vi "8-Tap 8-bit Camera with DRAM no Serial or Packing V4(FPGA).vi"() -> ()   [LabVIEW 2013]
doc: "This is the FPGA VI for the 10-Tap 8-Bit Camera with DRAM example. This example demonstrates how to acquire images from a 10-tap, 8-bit, extended configuration, Camera Link camera and transfer the images to the host. This example supports area scan and line scan cameras for both continuous and finite acquisitions.\n\nThis example also demonstrates the use of DRAM as a frame buffer for very high speed acquisitions. Data packing and flow-control are also employed to maximize use of the available DRAM and FIFOs in terms of both memory space and performance.\n\nAdditionally, the example demonstrates the serial server, which allows third-party camera configuration utilities to communicate with the camera using the Camera Link serial interface while this VI is running."
uses:
  <vilib>/rvi/DataTransferAndStorage/Container/XNode/niFpgaContainer.xnode
  <vilib>/Platform/TimedLoop/XDataNode/XDataNode.xnode
  <vilib>/Platform/TimedLoop/XDataNode/timing_clust.ctl
  <vilib>/Platform/TimedLoop/XDataNode/XDNodeRunTimeDep.lvlib
  <vilib>/Platform/TimedLoop/XDataNode/wakeup.ctl
  <vilib>/Platform/TimedLoop/XDataNode/nitl_modes.ctl
  <vilib>/eio/EIONode/EIONode.xnode
  <vilib>/rvi/eio/common/nirviEmuTemplateMethod_errors.vi
  <vilib>/rvi/FIFO/Fifo_Resource/nirvififoEmulationGetNumberOfElementsToRead.vi
  <vilib>/rvi/interface/RandomDataEmulation/nirviRandomDataFpgaReadWriteTemplate.vi
  <vilib>/rvi/FIFO/Fifo_Resource/nirvififoEmulationRead.vi
  <vilib>/rvi/FIFO/Fifo_Resource/nirvififoEmulationWrite.vi
  FPGA/Globals/Accumulated Sector Intensity.vi
  FPGA/Globals/Pixel Location Global.vi
  FPGA/Globals/Sector Parameter Global.vi
  <vilib>/rvi/FIFO/Fifo_Resource/nirvififoEmulationGetNumberOfElementsToWrite.vi
  Common/CL Data to Pixels/8 Tap 8-Bit.vi
  Common/CL Signal Mapping.ctl
  Common/CL Configuration.ctl
  FPGA/Sector/Accumulate/Sector Parameter Cluster.ctl
panel:
  in  "Right End Angle Duty Cycle":fxp<+,8,0>
  in  "Right Start Angle Duty Cycle":fxp<+,8,0>
  in  "Left End Angle Duty Cycle":fxp<+,8,0>
  in  "Left Start Angle Duty Cycle":fxp<+,8,0>
  in  "X Resolution":u16=1000
  in  "Y Resolution":u16=1000
  out "Analysis Ticks":u32
  out "Right Sector Edge":u8
  out "Left Sector Edge":u8
  in  "[Average BG Intensity]":u8[](array[numeric])=[0, 0, 0, 0, 0, 0, 0, 0, 0, 0, 0, 0, 0, 0, 0, 0, 0, 0, 0, 0, 0, 0, 0, 0, 0, 0, 0, 0, 0, 0, 0, 0]
  in  "Sector Threshold":u8
  in  "# of Frames to Average":u8
  in  "Sector Parameters Right":T1={"Start Angle"=0.0, "End Angle"=0.4708251953125, "Inner Radius"=309, "Outter Radius"=405, "Hinge X"=685, "Hinge Y"=527, "NumWingSectors"=8}
  in  "Sector Parameters Left":T1={"Start Angle"=0.65740966796875, "End Angle"=0.99468994140625, "Inner Radius"=309, "Outter Radius"=405, "Hinge X"=464, "Hinge Y"=534, "NumWingSectors"=8}
  in  "CL Config.Configuration":T2=enum."Full"
  in  "CL Config.Signal Mapping":T3=enum."Basler 10-tap"
  in  "CL Config.Line Scan":bool
  in  "CL Config.DVAL Active High":bool=TRUE
  in  "CL Config.LVAL Active High":bool=TRUE
  in  "CL Config.FVAL Active High":bool=TRUE
  in  "CL Config.Spare Active High":bool=TRUE
  in  "Acq Control.Line Scan Height":u32
  in  "Acq Control.Frames To Acq":u32
  in  "Acq Control.Acquire":bool
  in  "Acq Control.Cancel Acq":bool
  in  "Acq Control.Ignore DVAL":bool
  in  "Acq Control.Initialize":bool
  out "Acq Status.Acq In Progress":bool
  out "Acq Status.Clocks Per Line":u32
  out "Acq Status.Frames Acq'd":u32
  out "Acq Status.Lines Per Frame":u32
  out "Acq Status.DMA Write Timeout":bool
  out "Acq Status.Initialized":bool
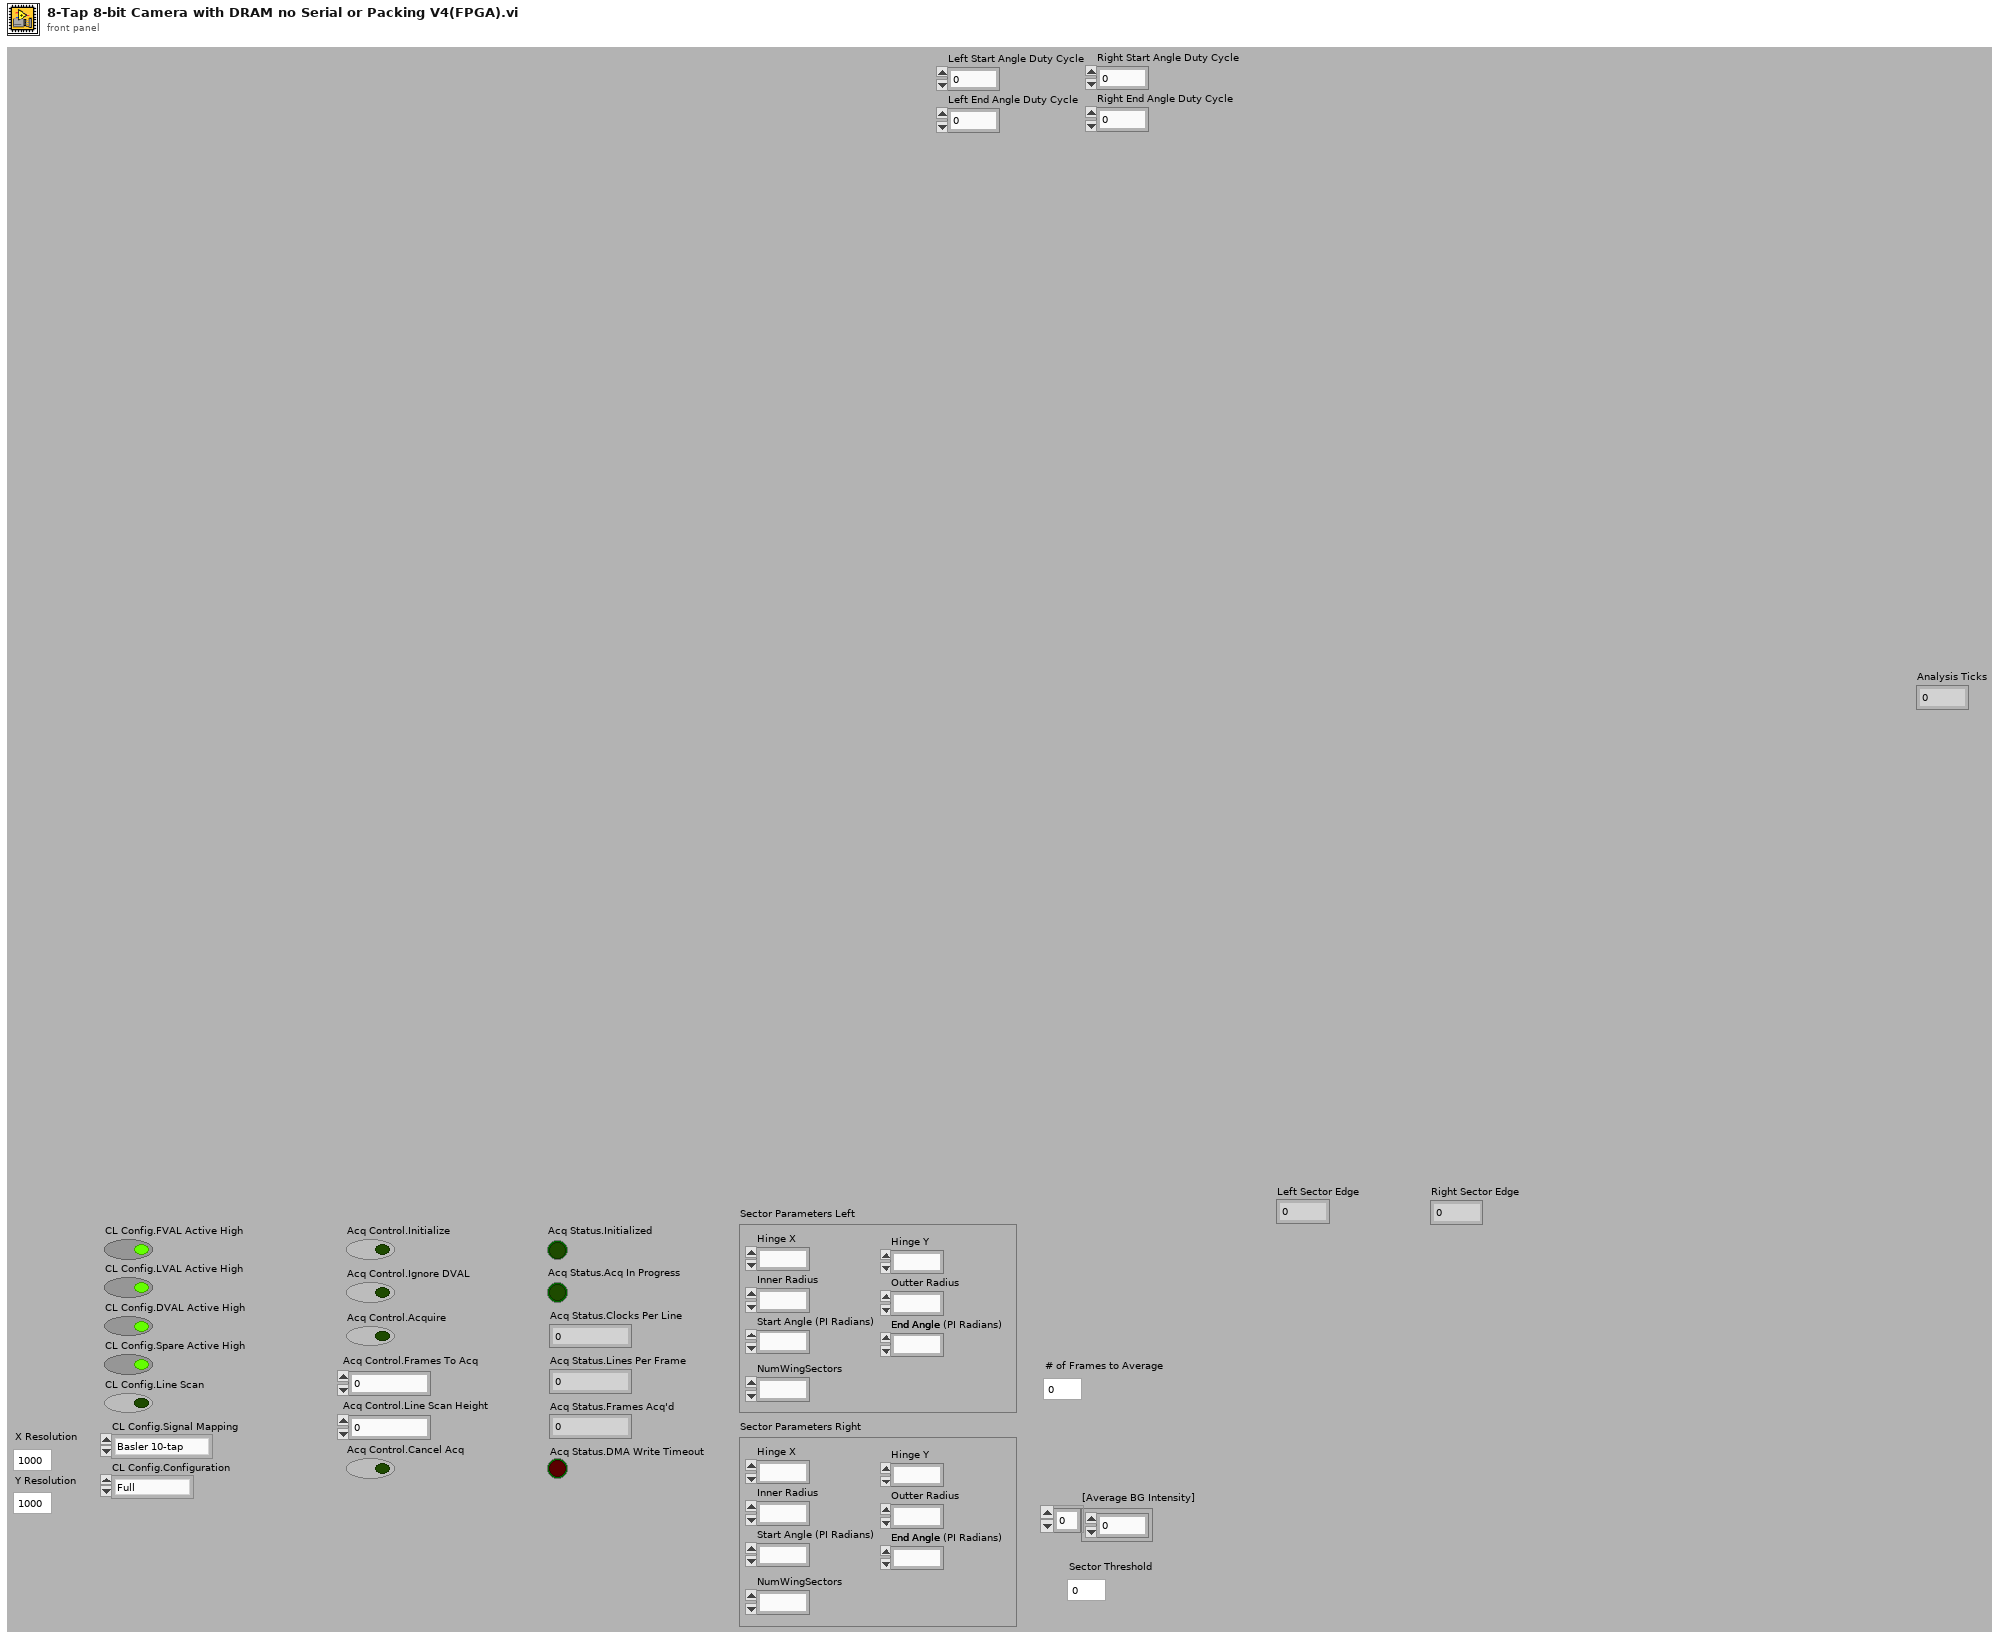
[diagram p1: front panel]
types:
  T1 = typedef "Sector Parameter Cluster.ctl" = cluster{"Start Angle":fxp<+/-,17,2>, "End Angle":fxp<+,17,3>, "Inner Radius":u16, "Outter Radius":u16, "Hinge X":u16, "Hinge Y":u16, "NumWingSectors":u8}
  T2 = typedef "CL Configuration.ctl" = enum8{"Base", "Medium", "Full"}
  T3 = typedef "CL Signal Mapping.ctl" = enum8{"Standard", "Basler 10-tap", "Vosskühler 10-tap"}
  T4 = typedef "XDNodeRunTimeDep.lvlib/timing_clust.ctl" = cluster{"Expected End [f-1]":u64, "Actual End [f-1]":u64, "Finished Late? [f-1]":bool, "Expected End [i-1]":u64, "Actual End [i-1]":u64, "Finished Late? [i-1]":bool, "Expected Start [i]":u64, "Actual Start [i]":u64, "Expected Start [f]":u64, "Actual Start [f]":u64, "Source Name":string, "Structure Name":string, "Period":i64, "Deadline":i64, "Offset":i64, "Start":i64, "Priority":i32, "Timeout":i32, "Mode":T5, "Wakeup Reason":T6, "Error":errorcluster, "Source Type":string, "Secondary Source Type":string, "Global End Time":u64, "Global Start Time":u64, "Frame Duration":u64, "Iteration Duration":u64, "Assigned CPU":i32, "I/O Scan Engine Mode":u32}
  T5 = typedef "XDNodeRunTimeDep.lvlib/nitl_modes.ctl" = enum32{"No Change", "Process missed periods, maintain original phase", "Discard missed periods, maintain original phase", "Process missed periods, ignore original phase", "Discard missed periods, ignore original phase"}
  T6 = typedef "XDNodeRunTimeDep.lvlib/wakeup.ctl" = enum32{"Normal", "Aborted", "Asynchronous wakeup", "Timing source error", "Timed loop error", "Timeout"}
  T7 = cluster{"Enables Valid":bool, "Frame Valid":bool, "Line Valid":bool, "Data Valid":bool}
  T8 = cluster{"Pixel 0":u8, "Pixel 1":u8, "Pixel 2":u8, "Pixel 3":u8, "Pixel 4":u8, "Pixel 5":u8, "Pixel 6":u8, "Pixel 7":u8}
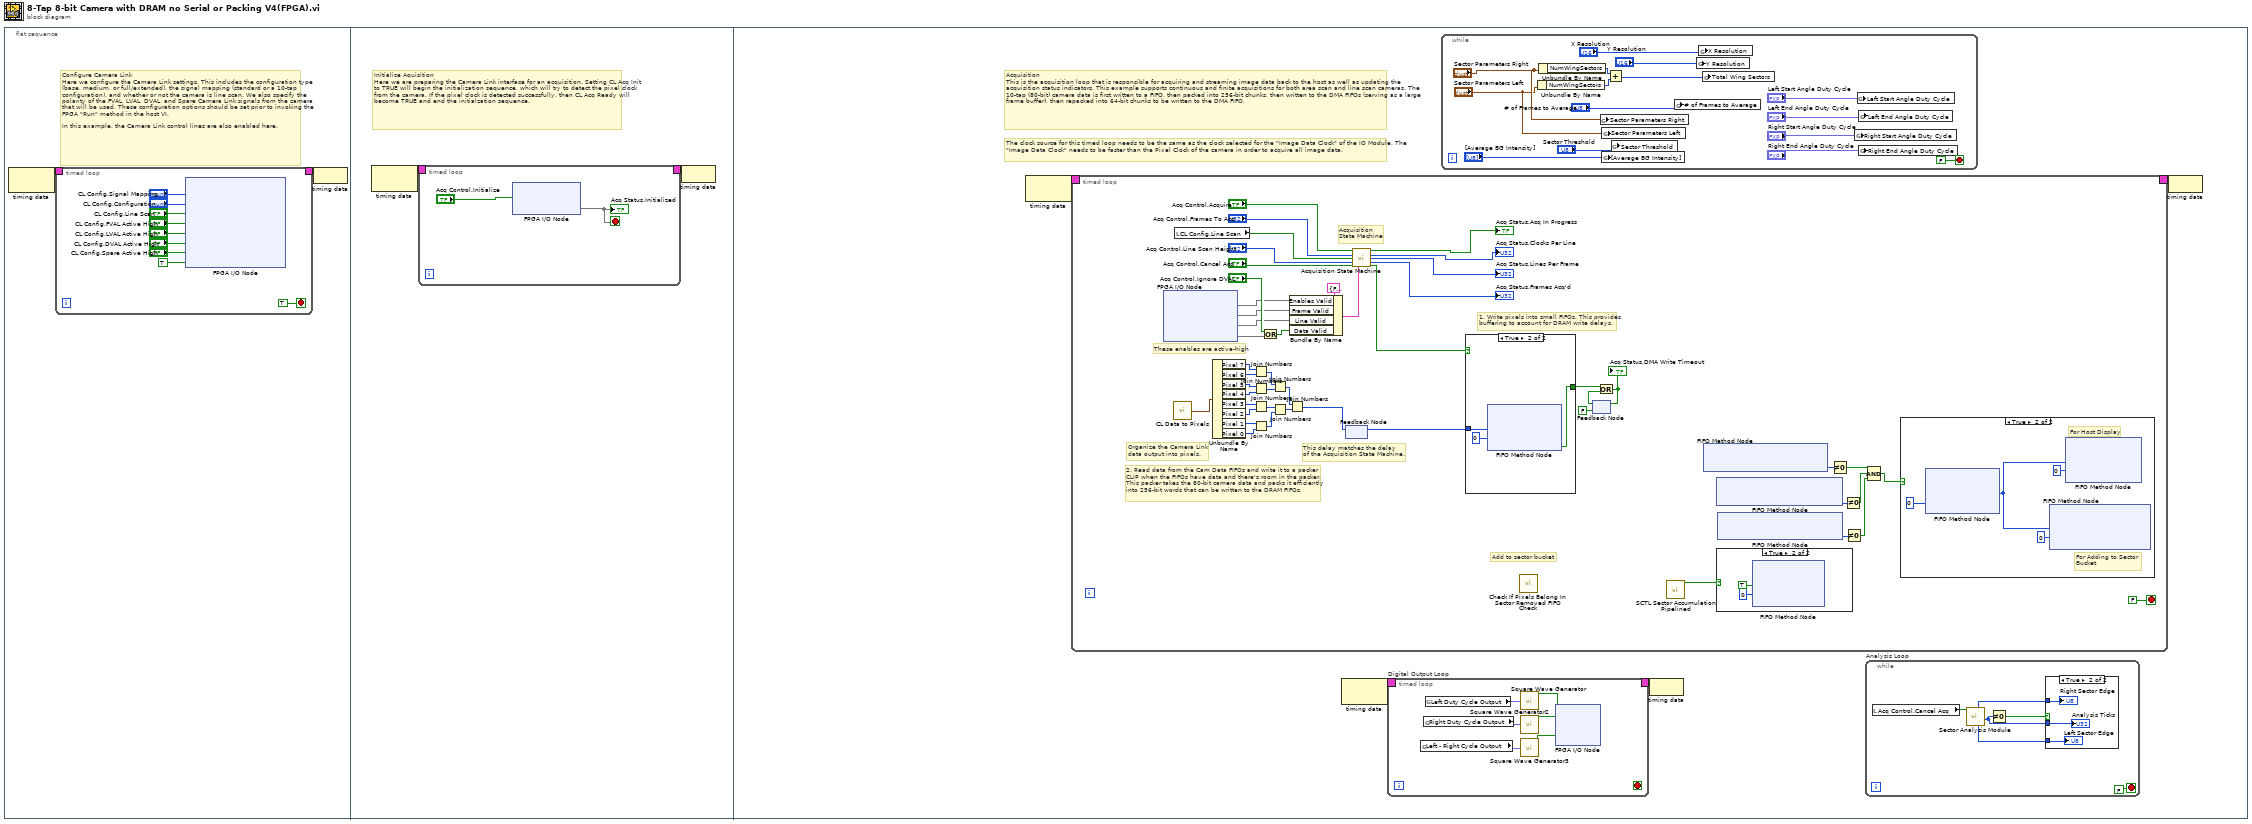
[diagram p0: block diagram]
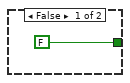
[diagram p5: hidden frame]
diagram:
  n1 = flat-sequence {
    frame #0 {
      # "Configure Camera Link\nHere we configure the Camera Link settings. This includes the configuration type (base, medium, or full/extended), the signal mapping (standard or a 10-tap configuration), and whether or not the camera is line scan. We also specify the polarity of the FVAL, LVAL, DVAL, and Spare Camera Link signals from the camera that will be used. These configuration options should be set prior to invoking the FPGA \"Run\" method in the host VI.\n\nIn this example, the Camera Link control lines are also enabled here."
      n2 = node-c288() -> (w2:T4)  [unwired: 1 in]
      n3 = timed-loop {
        timing: w2 -> [_]
        timing-out: [_] -> w1
        stop <- TRUE stop-if-true
        n4 = xnode "FPGA I/O Node"("CL Set Signal Mapping"="CL Config.Signal Mapping", "CL Set Configuration"="CL Config.Configuration", "CL Set Line Scan"="CL Config.Line Scan", "CL Set FVAL Active High"="CL Config.FVAL Active High", "CL Set LVAL Active High"="CL Config.LVAL Active High", "CL Set DVAL Active High"="CL Config.DVAL Active High", "CL Set Spare Active High"="CL Config.Spare Active High", "CL Control Enable"=TRUE ("IO Module\\CL Control Enable")) -> ()  [unwired: 8 in, 8 out]
      }
      n5 = node-c288(w1) -> ()
    }
    frame #1 {
      # "Initialize Aquisition\nHere we are preparing the Camera Link interface for an acquisition. Setting CL Acq Init to TRUE will begin the initialization sequence, which will try to detect the pixel clock from the camera. If the pixel clock is detected successfully, then CL Acq Ready will become TRUE and end the initialzation sequence."
      n6 = node-c288() -> (w17:T4)  [unwired: 1 out]
      n7 = timed-loop {
        timing: w17 -> [_]
        timing-out: [_] -> w16
        stop <- w18 stop-if-true
        n8 = xnode "FPGA I/O Node"("CL Acq Init"="Acq Control.Initialize") -> ("CL Acq Ready"=w18)  [unwired: 2 in, 2 out]
        "Acq Status.Initialized" <- w18
      }
      n9 = node-c288(w16) -> ()
    }
    frame #2 {
      # "The clock source for this timed loop needs to be the same as the clock selected for the \"Image Data Clock\" of the IO Module. The \"Image Data Clock\" needs to be faster than the Pixel Clock of the camera in order to acquire all image data."
      # "Acquisition\nThis is the acquisition loop that is responsible for acquiring and streaming image data back to the host as well as updating the acquisition status indicators. This example supports continuous and finite acquisitions for both area scan and line scan cameras. The 10-tap (80-bit) camera data is first written to a FIFO, then packed into 256-bit chunks, then written to the DMA FIFOs (serving as a large frame buffer), then repacked into 64-bit chunks to be written to the DMA FIFO."
      n10 = node-c288() -> (w27:T4)  [unwired: 1 in]
      n11 = timed-loop {
        timing: w27 -> [_]
        timing-out: [_] -> w26
        stop <- FALSE stop-if-true
        # "Add to sector bucket"
        # "These enables are active-high"
        # "Acquisition\nState Machine"
        # "2. Read data from the Cam Data FIFOs and write it to a packer\nCLIP when the FIFOs have data and there's room in the packer.\nThis packer takes the 80-bit camera data and packs it efficiently\ninto 256-bit words that can be written to the DRAM FIFOs."
        # "Organize the Camera Link\ndata output into pixels."
        # "This delay matches the delay\nof the Acquisition State Machine."
        # "1. Write pixels into small FIFOs. This provides\nbuffering to account for DRAM write delays."
        n12 = xnode "FPGA I/O Node"() -> ("CL Output Valid"=w69, "CL Frame Valid"=w70, "CL Line Valid"=w71, "CL Data Valid"=w74)  [unwired: 4 in, 4 out]
        n13 = call-poly "CL Data to Pixels.vi"() -> ("Pixels"=w51:T8)  [unwired: 1 in]
        n14 = local read "CL Config.Line Scan"() -> (w77:bool)
        n15 = Unbundle By Name(w51) -> ("Pixel 7"=w65:u8, "Pixel 6"=w64:u8, "Pixel 5"=w63:u8, "Pixel 4"=w62:u8, "Pixel 3"=w61:u8, "Pixel 2"=w60:u8, "Pixel 1"=w59:u8, "Pixel 0"=w58:u8)
        n16 = Join Numbers(hi=w65, lo=w64) -> ((hi.lo)=w56:u16)
        n17 = Join Numbers(hi=w63, lo=w62) -> ((hi.lo)=w55:u16)
        n18 = Join Numbers(hi=w61, lo=w60) -> ((hi.lo)=w54:u16)
        n19 = Join Numbers(hi=w59, lo=w58) -> ((hi.lo)=w57:u16)
        n20 = Or(x="Acq Control.Ignore DVAL", y=w74) -> (x .or. y?=w75:bool)
        n21 = Join Numbers(hi=w56, lo=w55) -> ((hi.lo)=w53:u32)
        n22 = Join Numbers(hi=w54, lo=w57) -> ((hi.lo)=w52:u32)
        n23 = Join Numbers(hi=w53, lo=w52) -> ((hi.lo)=w50:u64)
        n24 = Bundle By Name(cluster=T7 {"Enables Valid"=FALSE, "Frame Valid"=FALSE, "Line Valid"=FALSE, "Data Valid"=FALSE} ("Enables"), "Enables Valid"=w69, "Frame Valid"=w70, "Line Valid"=w71, "Data Valid"=w75) -> (w72:T7)
        n25 = feedback #1() -> (w94:u64)  [unwired: 1 in]
        n26 = feedback-in #1(w50) -> ()
        n27 = call "Acquisition State Machine.vi"("Acquire"="Acq Control.Acquire", "Frames to Acquire"="Acq Control.Frames To Acq", "Line Scan"=w77, "Line Scan Height"="Acq Control.Line Scan Height", "Cancel Acq"="Acq Control.Cancel Acq", "Enables"=w72) -> ("Acq In Progress"=→"Acq Status.Acq In Progress":bool, "Num Clocks Per Line"=→"Acq Status.Clocks Per Line":u32, "Num Lines Per Frame"=→"Acq Status.Lines Per Frame":u32, "Num Frames Acq'd"=→"Acq Status.Frames Acq'd":u32, "Capture Cycle"=w87:bool)  [unwired: 4 in, 1 out]
        n28 = case shown="True" w87 {
          tunnel: [FALSE ("Timed Out?") w103] -> w92
          tunnel: w94 -> [_ w104]
          frame False {
          }
          frame True {
            n29 = xnode ("FIFO Method Node")("Element"=w104, "Timeout"=0) -> ("Timed Out?"=w103:bool)  [unwired: 1 in, 1 out]
          }
        }
        n30 = call "Check If Pixels Belong In Sector Removed FIFO Check.vi"() -> ()  [unwired: 11 in, 1 out]
        n31 = feedback #2(FALSE) -> (w91:bool)
        n32 = Or(x=w92, y=w91) -> (x .or. y?=w90:bool)
        "Acq Status.DMA Write Timeout" <- w90
        n33 = feedback-in #2(w90) -> ()
        n34 = call "SCTL Sector Accumulation Pipelined.vi"() -> ("New Data?"=w47:bool)  [unwired: 11 in]
        n35 = xnode ("FIFO Method Node")() -> ("Number of Elements to Read"=w89:u32)  [unwired: 1 in, 1 out]
        n36 = xnode ("FIFO Method Node")() -> ("Number of Elements to Write"=w81:u32)  [unwired: 1 in, 1 out]
        n37 = case shown="True" w47 {
          frame False {
          }
          frame True {
            n38 = xnode ("FIFO Method Node")("Element"=TRUE, "Timeout"=0) -> ()  [unwired: 1 in, 2 out]
          }
        }
        n39 = xnode ("FIFO Method Node")() -> ("Number of Elements to Write"=w80:u32)  [unwired: 1 in, 1 out]
        n40 = Not Equal To 0?(x=w89) -> (x != 0?=w49:bool)
        n41 = Not Equal To 0?(x=w81) -> (x != 0?=w82:bool)
        n42 = Not Equal To 0?(x=w80) -> (x != 0?=w79:bool)
        n43 = Compound Arithmetic op=AND(w49, w82, w79) -> (w48:bool)
        n44 = case shown="True" w48 {
          frame False {
          }
          frame True {
            # "For Adding to Sector \nBucket"
            # "For Host Display"
            n45 = xnode ("FIFO Method Node")("Timeout"=0) -> ("Element"=w97:u64)  [unwired: 1 in, 2 out]
            n46 = xnode ("FIFO Method Node")("Element"=w97, "Timeout"=0) -> ()  [unwired: 1 in, 2 out]
            n47 = xnode ("FIFO Method Node")("Element"=w97, "Timeout"=0) -> ()  [unwired: 1 in, 2 out]
          }
        }
      }
      n48 = node-c288() -> (w25:T4)  [unwired: 1 in]
      n49 = timed-loop "Digital Output Loop" {
        timing: w25 -> [_]
        timing-out: [_] -> w24
        stop <- _ stop-if-true
        n50 = global read "Sector Parameter Global.vi" "Left - Right Cycle Output"() -> (w40:fxp<+,8,0>)
        n51 = global read "Sector Parameter Global.vi" "Right Duty Cycle Output"() -> (w41:fxp<+,8,0>)
        n52 = global read "Sector Parameter Global.vi" "Left Duty Cycle Output"() -> (w42:fxp<+,8,0>)
        n53 = call "Square Wave Generator"("duty cycle (periods)"=w42) -> ("square wave out"=w39:bool)  [unwired: 14 in]
        n54 = call "Square Wave Generator2"("duty cycle (periods)"=w41) -> ("square wave out"=w38:bool)  [unwired: 14 in]
        n55 = call "Square Wave Generator3"("duty cycle (periods)"=w40) -> ("square wave out"=w37:bool)  [unwired: 14 in]
        n56 = xnode "FPGA I/O Node"("TTL 0"=w39, "TTL 1"=w38, "TTL 2"=w37) -> ()  [unwired: 3 in, 3 out]
      }
      n57 = while {
        stop <- FALSE stop-if-true
        n58 = Unbundle By Name("Sector Parameters Left") -> ("NumWingSectors"=w121:u8)
        n59 = Unbundle By Name("Sector Parameters Right") -> ("NumWingSectors"=w122:u8)
        n60 = global write "Sector Parameter Global.vi" "Sector Parameters Right"("Sector Parameters Right") -> ()
        n61 = global write "Sector Parameter Global.vi" "Sector Parameters Left"("Sector Parameters Left") -> ()
        n62 = global write "Sector Parameter Global.vi" "[Average BG Intensity]"("[Average BG Intensity]") -> ()
        n63 = Add(x=w122, y=w121) -> (x+y=w120:u8)
        n64 = global write "Sector Parameter Global.vi" "Sector Threshold"("Sector Threshold") -> ()
        n65 = global write "Pixel Location Global.vi" "# of Frames to Average"("# of Frames to Average") -> ()
        n66 = global write "Pixel Location Global.vi" "Y Resolution"("Y Resolution") -> ()
        n67 = global write "Pixel Location Global.vi" "X Resolution"("X Resolution") -> ()
        n68 = global write "Accumulated Sector Intensity.vi" "Total Wing Sectors"(w120) -> ()
        n69 = global write "Sector Parameter Global.vi" "Right Start Angle Duty Cycle"("Right Start Angle Duty Cycle") -> ()
        n70 = global write "Sector Parameter Global.vi" "Left Start Angle Duty Cycle"("Left Start Angle Duty Cycle") -> ()
        n71 = global write "Sector Parameter Global.vi" "Left End Angle Duty Cycle"("Left End Angle Duty Cycle") -> ()
        n72 = global write "Sector Parameter Global.vi" "Right End Angle Duty Cycle"("Right End Angle Duty Cycle") -> ()
      }
      n73 = node-c288(w24) -> ()
      n74 = while "Analysis Loop" {
        stop <- FALSE stop-if-true
        n75 = local read "Acq Control.Cancel Acq"() -> (w32:bool)
        n76 = call "Sector Analysis Module.vi"("Canceled?"=w32) -> ("Analysis Ticks"=w31:u32, "Left Sector Edge"=w28:u8, "Right Sector Edge"=w29:u8)  [unwired: 6 in, 2 out]
        n77 = Not Equal To 0?(x=w31) -> (x != 0?=w30:bool)
        n78 = case shown="True" w30 {
          tunnel: w31 -> [_ w36]
          tunnel: w29 -> [_ w35]
          tunnel: w28 -> [_ w34]
          frame False {
          }
          frame True {
            "Analysis Ticks" <- w36
            "Right Sector Edge" <- w35
            "Left Sector Edge" <- w34
          }
        }
      }
      n79 = node-c288(w26) -> ()
    }
  }
